vi "take numeric string values out to 001 place holder.vi"(11 "String number out to .001":string) -> (3 "formated result":string)   [LabVIEW 2010]
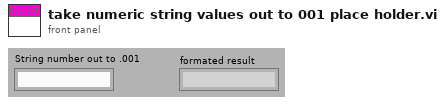
[diagram p1: front panel]
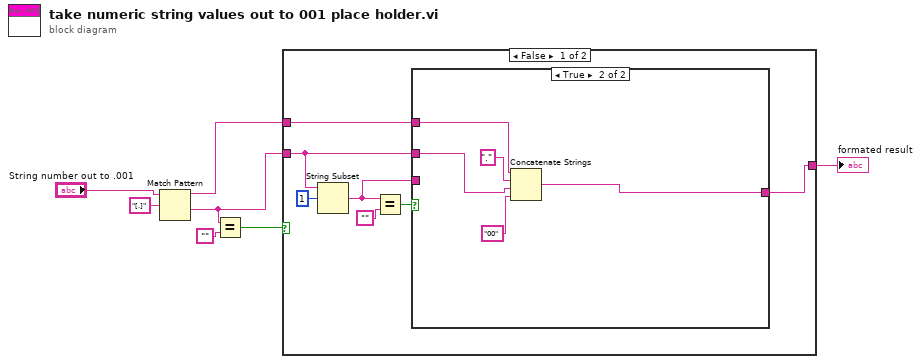
[diagram p0: block diagram]
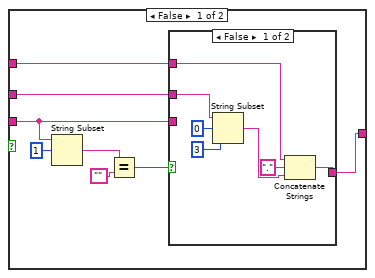
[diagram p2: hidden frame]
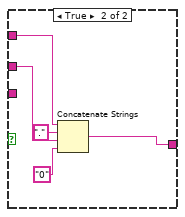
[diagram p3: hidden frame]
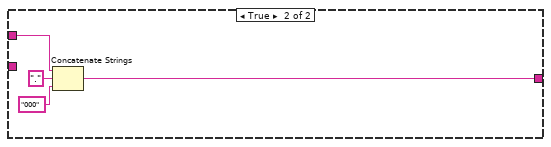
[diagram p4: hidden frame]
diagram:
  n1 = Match Pattern(string="String number out to .001", regular expression="[.]") -> (before substring=w1:string, after substring=w2:string)  [unwired: 1 in, 2 out]
  n2 = Equal?(x=w2, y="") -> (x = y?=w4:bool)
  n3 = case shown="False" w4 {
    tunnel: [w11 w41] -> w3
    tunnel: w1 -> [w8 w40]
    tunnel: w2 -> [w9 _]
    frame False {
      n4 = String Subset(string=w9, offset (0)=1) -> (substring=w10:string)  [unwired: 1 in]
      n5 = Equal?(x=w10, y="") -> (x = y?=w12:bool)
      n6 = case shown="True" w12 {
        tunnel: w9 -> [w16 w35]
        tunnel: [w17 w38] -> w11
        tunnel: w10 -> [w18 _]
        tunnel: w8 -> [w15 w37]
        frame False {
          n7 = String Subset(string=w18, offset (0)=1) -> (substring=w22:string)  [unwired: 1 in]
          n8 = Equal?(x=w22, y="") -> (x = y?=w19:bool)
          n9 = case shown="False" w19 {
            tunnel: w18 -> [_ _]
            tunnel: [w26 w33] -> w17
            tunnel: w16 -> [w28 w32]
            tunnel: w15 -> [w23 w30]
            frame False {
              n10 = String Subset(string=w28, offset (0)=0, length (rest)=3 ("length (rest)")) -> (substring=w25:string)
              n11 = Concatenate Strings(w23, "." ("string"), w25) -> (w26:string)
            }
            frame True {
              n12 = Concatenate Strings(w30, "." ("string"), w32, "0" ("string")) -> (w33:string)
            }
          }
        }
        frame True {
          n13 = Concatenate Strings(w37, "." ("string"), w35, "00" ("string")) -> (w38:string)
        }
      }
    }
    frame True {
      n14 = Concatenate Strings(w40, "." ("string"), "000" ("string")) -> (w41:string)
    }
  }
  "formated result" <- w3
